vi "sub Error Popup.vi"(0 "Error Message":string, 3 "error in":errorcluster, 4 "Console Ref":refnum<vi>) -> (5 "Continue Out":bool, 6 "Quit Out":bool, 7 "error out":errorcluster)   [LabVIEW 2025]
doc: "When a VISA error occurs in the main GUI demo program, this VI pops-up to show the VISA error message. The message is also appended to the Command Logging text box. The user may select to Continue or Quit the GUI demo program."
panel:
  out "Err Descr":string
  out "code":i32
  out "status":bool caption="ERROR"
  in  "Quit":bool
  in  "Continue":bool
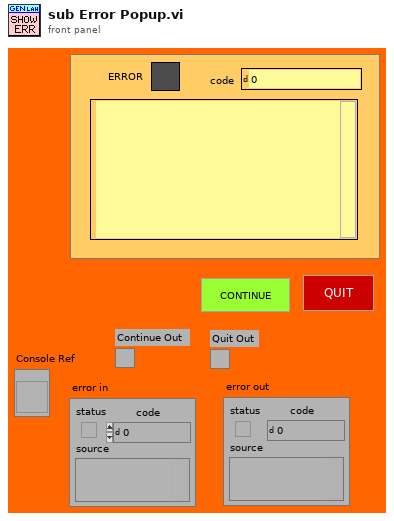
[diagram p1: front panel]
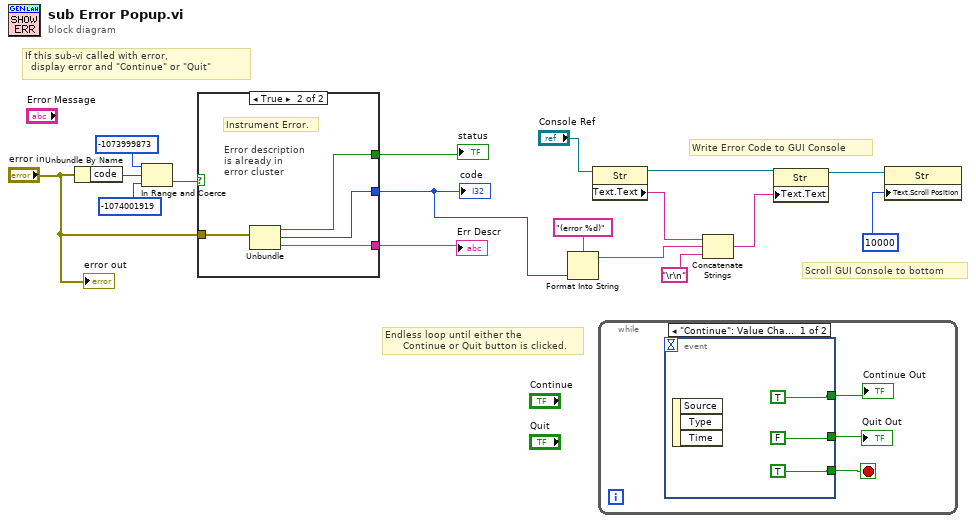
[diagram p0: block diagram]
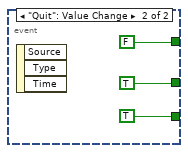
[diagram p2: hidden frame]
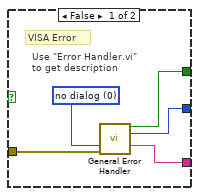
[diagram p3: hidden frame]
diagram:
  # "Scroll GUI Console to bottom"
  # "Endless loop until either the \n      Continue or Quit button is clicked."
  # "Write Error Code to GUI Console"
  # "If this sub-vi called with error,\n  display error and \"Continue\" or \"Quit\""
  n1 = Unbundle By Name("error in") -> ("code"=w14:i32)
  n2 = In Range and Coerce(upper limit=-1073999873 ("code"), x=w14, lower limit=-1074001919 ("code")) -> (In Range?=w13:bool)  [unwired: 1 out]
  n3 = case shown="True" w13 {
    tunnel: "error in" -> [w22 w26]
    tunnel: [w20 w23] -> w17
    tunnel: [w19 w24] -> w1
    tunnel: [w18 w25] -> w16
    frame False {
      w21 = u16 0 items=["no dialog", "OK message", "continue or stop message"] ("type of dialog (OK msg:1)")
      # "Use \"Error Handler.vi\"\nto get description"
      # "VISA Error"
      n4 = call <vilib>:"General Error Handler.vi"("type of dialog (OK msg:1)"=w21, "error in (no error)"=w22) -> ("error?"=w18:bool, "code out"=w19:i32, "message"=w20:string)  [unwired: 9 in, 2 out]
    }
    frame True {
      # "Error description\nis already in\nerror cluster"
      # "Instrument Error."
      n5 = Unbundle(w26) -> ("status"=w25:bool, "code"=w24:i32, "source"=w23:string)
    }
  }
  "status" <- w16
  "code" <- w1
  "Err Descr" <- w17
  n6 = Format Into String(format string="(error %d)", w1) -> (resulting string=w4:string)  [unwired: 2 in, 1 out]
  n7 = property class="Str"(reference="Console Ref") -> (reference out=w10:refnum<vi>, "Text.Text"=w11:string)  [unwired: 1 in, 1 out]
  n8 = while {
    stop <- w27 stop-if-true
    n9 = event shown="[0] \"Continue\": Value Change" {
      selector: _ -> [_ _]
      dyn-events: _ -> [_ _]
      timeout: _ -> [_ _]
      tunnel: [TRUE FALSE] -> w29
      tunnel: [FALSE TRUE] -> w28
      tunnel: [TRUE TRUE] -> w27
      event "Continue": Value Change {
        n10 = event-data() -> ()  [unwired: 1 in, 3 out]
      }
      event "Quit": Value Change {
        n11 = event-data() -> ()  [unwired: 1 in, 3 out]
      }
    }
    "Continue Out" <- w29
    "Quit Out" <- w28
  }
  n12 = Concatenate Strings(w11, w4, "\r\n") -> (w9:string)
  n13 = property class="Str"(reference=w10, "Text.Text"=w9) -> (reference out=w8:refnum<vi>)  [unwired: 1 in, 1 out]
  n14 = property class="Str"(reference=w8, "Text.Scroll Position"=u32 10000) -> ()  [unwired: 1 in, 2 out]
  "error out" <- "error in"
